vi "Convert Absolute to Relative Coords.vi"(7 "Relative Movement Type":T1, 8 "error in (no error)":errorcluster, 9 "Relative Object Name":string, 10 "Y":i32, 11 "X":i32) -> (0 "error out":errorcluster, 2 "Relative Y":i32, 3 "Relative X":i32)   [LabVIEW 2020, in "MacroAssert.lvlib" / "Mouse Action.lvclass"]
uses:
  Mouse Action.lvclass
  Mouse Action.lvclass/Mouse Action.ctl
  SubVIs/Win Util/Win Util.lvlib
  MacroAssert.lvlib
  Relative Movement Type.ctl
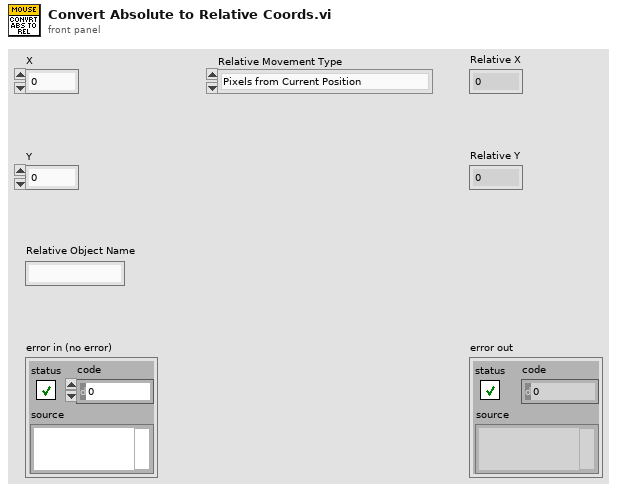
[diagram p1: front panel]
types:
  T1 = typedef "MacroAssert.lvlib/Mouse Action.lvclass/Relative Movement Type.ctl" = enum16{"Pixels from Current Position", "Pixels from Top-Left of Control", "Pixels from Top-Left of Window", "Percentage from Top-Left of Control", "Percentage from Top-Left of Window", "Percentage from Top-Left of Screen"}
  T2 = typedef "LVPositionTypeDef.ctl" = cluster{"Left":i32, "Top":i32}
  T3 = typedef "LVBoundsTypeDef.ctl" = cluster{"Width":u32, "Height":u32}
  T4 = typedef "LVPointTypeDef.ctl" = cluster{"Horizontal":i16, "Vertical":i16}
  T5 = typedef "MacroAssert.lvlib/Win Util.lvlib/Window Refnum.ctl" = u64
  T6 = cluster{"left":i16, "top":i16, "right":i16, "bottom":i16}
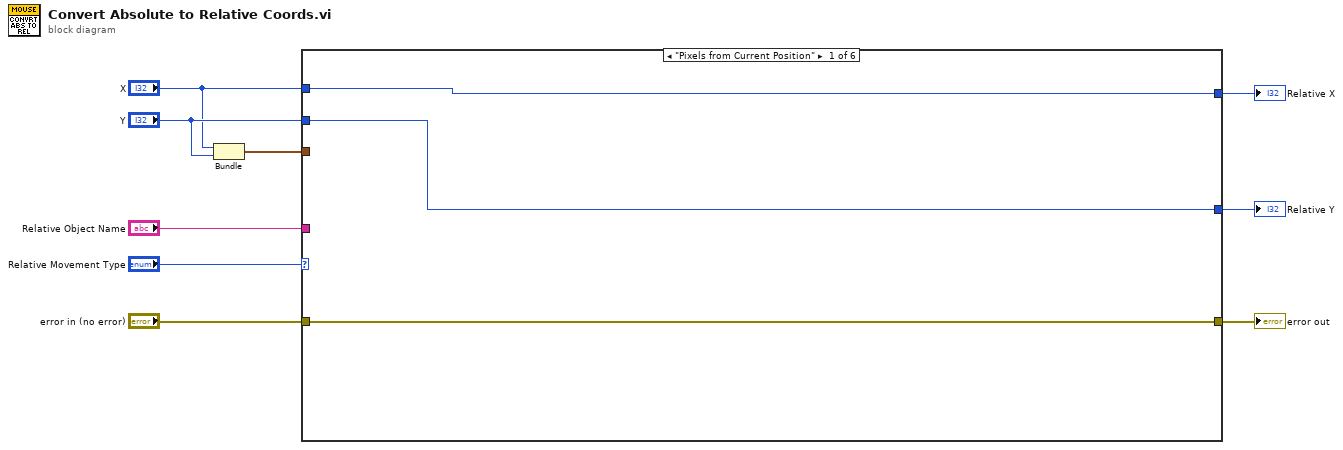
[diagram p0: block diagram]
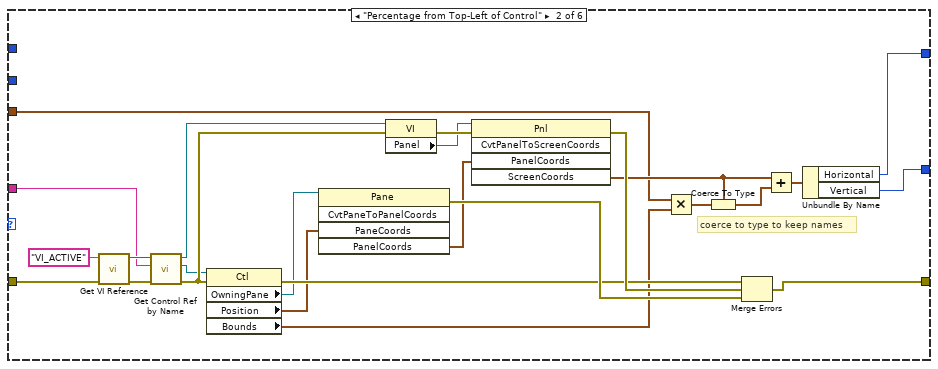
[diagram p2: hidden frame]
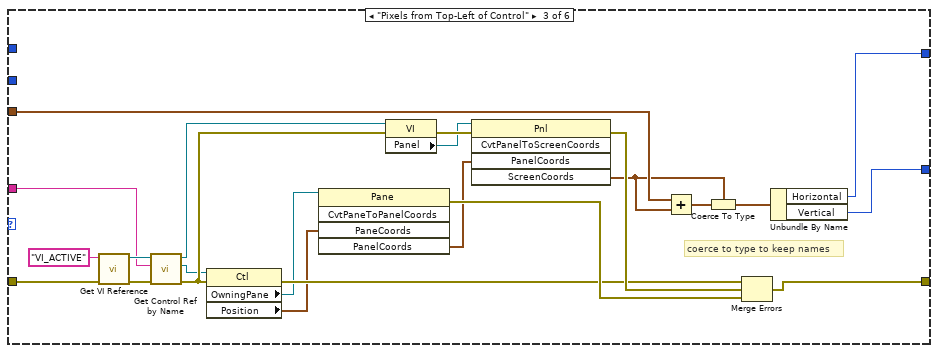
[diagram p3: hidden frame]
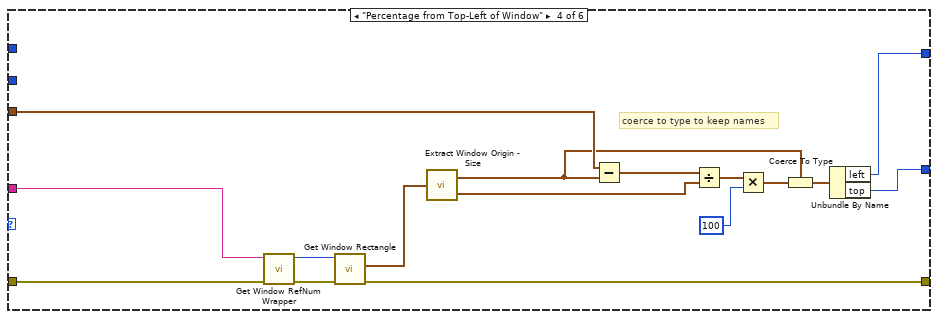
[diagram p4: hidden frame]
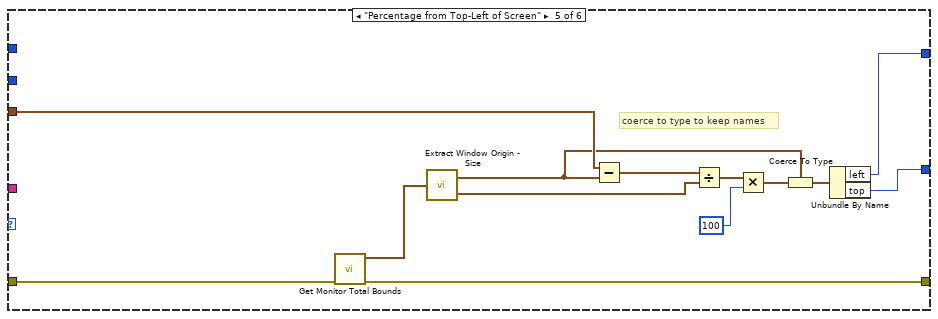
[diagram p5: hidden frame]
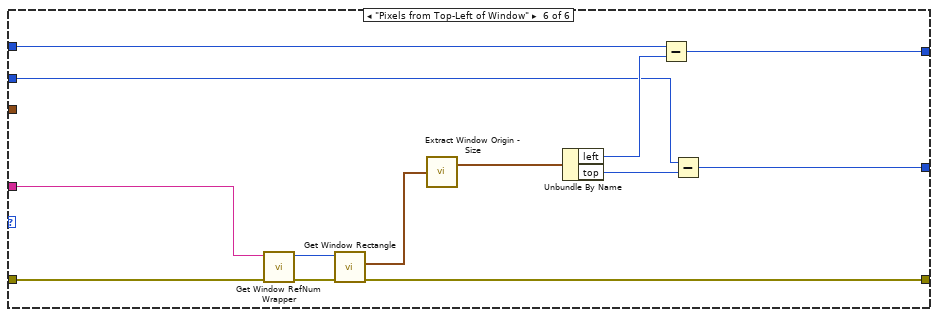
[diagram p6: hidden frame]
diagram:
  n1 = Bundle("X"="X", "Y"="Y") -> (w1:cluster{"X":i32, "Y":i32})  [unwired: 1 in]
  n2 = case shown="\"Pixels from Current Position\"" "Relative Movement Type" {
    tunnel: "error in (no error)" -> [w10 w33 w56 w71 w77 w100]
    tunnel: [w10 w25 w48 w70 w86 w99] -> w8
    tunnel: "Relative Object Name" -> [_ w30 w53 w68 _ w96]
    tunnel: [w11 w19 w46 w76 w89 w90] -> w4
    tunnel: [w12 w18 w45 w75 w88 w93] -> w5
    tunnel: w1 -> [_ w17 w44 w69 w85 _]
    tunnel: "Y" -> [w11 _ _ _ _ w91]
    tunnel: "X" -> [w12 _ _ _ _ w94]
    frame "Pixels from Current Position" {
    }
    frame "Percentage from Top-Left of Control" {
      # "coerce to type to keep names"
      n3 = call "Get VI Reference.vi"("error in (no error)"=w33, "VI Name"="VI_ACTIVE") -> ("error out"=w32:errorcluster, "VI Ref"=w31:refnum<vi>)  [unwired: 8 in]
      n4 = call "Get Control Ref by Name.vi"("error in (no error)"=w32, "Name"=w30, "VI Ref"=w31) -> ("error out"=w35:errorcluster, "Ctl Ref"=w29:refnum<vi>, "VI Ref out"=w28:refnum<vi>)  [unwired: 6 in]
      n5 = property class="Ctl"(reference=w29, error in=w35) -> (error out=w26:errorcluster, "OwningPane"=w15:refnum<vi>, "Position"=w14:T2, "Bounds"=w24:T3)  [unwired: 1 out]
      n6 = invoke class="Pane" method="CvtPaneToPanelCoords"(reference=w15, "PaneCoords"=w14) -> (error out=w36:errorcluster, "PanelCoords"=w16:T4)  [unwired: 3 in, 3 out]
      n7 = property class="VI"(reference=w28, error in=w35) -> (error out=w34:errorcluster, "Panel"=w27:refnum<vi>)  [unwired: 1 out]
      n8 = invoke class="Pnl" method="CvtPanelToScreenCoords"(reference=w27, error in=w34, "PanelCoords"=w16) -> (error out=w37:errorcluster, "ScreenCoords"=w21:T4)  [unwired: 2 in, 3 out]
      n9 = Multiply(x=w17, y=w24) -> (x*y=w23:T3)
      n10 = Coerce To Type(0:w23, 1:w21) -> (2:w22:T4)
      n11 = Merge Errors(w26, w37, w36) -> (w25:errorcluster)
      n12 = Add(x=w21, y=w22) -> (x+y=w20:T4)
      n13 = Unbundle By Name(w20) -> ("Horizontal"=w18:i16, "Vertical"=w19:i16)
    }
    frame "Pixels from Top-Left of Control" {
      # "coerce to type to keep names"
      n14 = call "Get VI Reference.vi"("error in (no error)"=w56, "VI Name"="VI_ACTIVE") -> ("error out"=w55:errorcluster, "VI Ref"=w54:refnum<vi>)  [unwired: 8 in]
      n15 = call "Get Control Ref by Name.vi"("error in (no error)"=w55, "Name"=w53, "VI Ref"=w54) -> ("error out"=w58:errorcluster, "Ctl Ref"=w52:refnum<vi>, "VI Ref out"=w51:refnum<vi>)  [unwired: 6 in]
      n16 = property class="Ctl"(reference=w52, error in=w58) -> (error out=w49:errorcluster, "OwningPane"=w42:refnum<vi>, "Position"=w41:T2)  [unwired: 1 out]
      n17 = invoke class="Pane" method="CvtPaneToPanelCoords"(reference=w42, "PaneCoords"=w41) -> (error out=w59:errorcluster, "PanelCoords"=w43:T4)  [unwired: 3 in, 3 out]
      n18 = property class="VI"(reference=w51, error in=w58) -> (error out=w57:errorcluster, "Panel"=w50:refnum<vi>)  [unwired: 1 out]
      n19 = invoke class="Pnl" method="CvtPanelToScreenCoords"(reference=w50, error in=w57, "PanelCoords"=w43) -> (error out=w60:errorcluster, "ScreenCoords"=w40:T4)  [unwired: 2 in, 3 out]
      n20 = Add(x=w44, y=w40) -> (x+y=w47:cluster{i32, i32})
      n21 = Coerce To Type(0:w47, 1:w40) -> (2:w39:T4)
      n22 = Merge Errors(w49, w60, w59) -> (w48:errorcluster)
      n23 = Unbundle By Name(w39) -> ("Horizontal"=w45:i16, "Vertical"=w46:i16)
    }
    frame "Percentage from Top-Left of Window" {
      # "coerce to type to keep names"
      n24 = call "Get Window RefNum Wrapper.vi"("error in (no error)"=w71, "Window Name"=w68) -> ("error out"=w73:errorcluster, "window refnum"=w74:T5)  [unwired: 8 in]
      n25 = call "Get Window Rectangle.vi"("error in (no error)"=w73, "window refnum (NaWR)"=w74) -> ("error out"=w70:errorcluster, "window rect"=w72:T6)  [unwired: 7 in, 1 out]
      n26 = call "Extract Window Origin - Size.vi"("window rect"=w72) -> ("window origin"=w62:cluster{"left":i16, "top":i16}, "window size"=w63:cluster{"Width":i16, "Height":i16})
      n27 = Subtract(x=w69, y=w62) -> (x-y=w64:cluster{i32, i32})
      n28 = Divide(x=w64, y=w63) -> (x/y=w66:cluster{dbl, dbl})
      n29 = Multiply(x=w66, y=100) -> (x*y=w65:cluster{dbl, dbl})
      n30 = Coerce To Type(0:w65, 1:w62) -> (2:w61:cluster{"left":i16, "top":i16})
      n31 = Unbundle By Name(w61) -> ("left"=w75:i16, "top"=w76:i16)
    }
    frame "Percentage from Top-Left of Screen" {
      # "coerce to type to keep names"
      n32 = call "Get Monitor Total Bounds.vi"("error in (no error)"=w77) -> ("error out"=w86:errorcluster, "window rect"=w87:T6)  [unwired: 9 in]
      n33 = call "Extract Window Origin - Size.vi"("window rect"=w87) -> ("window origin"=w79:cluster{"left":i16, "top":i16}, "window size"=w80:cluster{"Width":i16, "Height":i16})
      n34 = Subtract(x=w85, y=w79) -> (x-y=w81:cluster{i32, i32})
      n35 = Divide(x=w81, y=w80) -> (x/y=w83:cluster{dbl, dbl})
      n36 = Multiply(x=w83, y=100) -> (x*y=w82:cluster{dbl, dbl})
      n37 = Coerce To Type(0:w82, 1:w79) -> (2:w78:cluster{"left":i16, "top":i16})
      n38 = Unbundle By Name(w78) -> ("left"=w88:i16, "top"=w89:i16)
    }
    frame "Pixels from Top-Left of Window" {
      n39 = call "Get Window RefNum Wrapper.vi"("error in (no error)"=w100, "Window Name"=w96) -> ("error out"=w101:errorcluster, "window refnum"=w102:T5)  [unwired: 8 in]
      n40 = call "Get Window Rectangle.vi"("error in (no error)"=w101, "window refnum (NaWR)"=w102) -> ("error out"=w99:errorcluster, "window rect"=w98:T6)  [unwired: 7 in, 1 out]
      n41 = call "Extract Window Origin - Size.vi"("window rect"=w98) -> ("window origin"=w97:cluster{"left":i16, "top":i16})  [unwired: 1 out]
      n42 = Unbundle By Name(w97) -> ("left"=w95:i16, "top"=w92:i16)
      n43 = Subtract(x=w94, y=w95) -> (x-y=w93:i32)
      n44 = Subtract(x=w91, y=w92) -> (x-y=w90:i32)
    }
  }
  "error out" <- w8
  "Relative X" <- w5
  "Relative Y" <- w4
